vi "BNNN.vi"(11 "Variables and Memory in":T1 {"GFX" format="%02x"}) -> (3 "Variables and Memory out":T1 {"GFX" format="%02x"})   [LabVIEW 2021]
uses:
  Controls/ClusterF.ctl
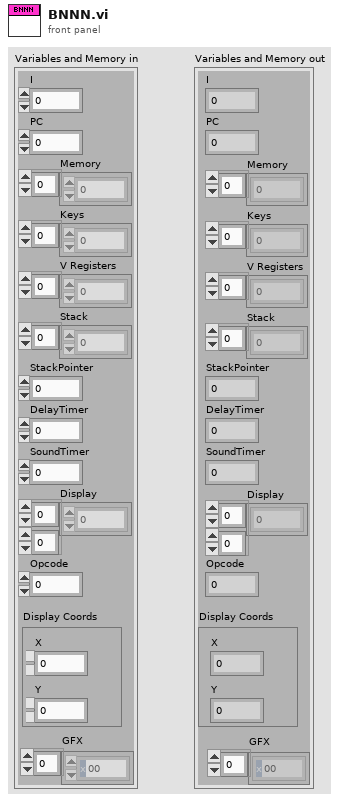
[diagram p1: front panel]
types:
  T1 = typedef "ClusterF.ctl" = cluster{"I":u16, "PC":u16, "Memory":u8[], "Keys":u8[], "V Registers":u8[], "Stack":u16[], "StackPointer":u16, "DelayTimer":u8, "SoundTimer":u8, "Display":u8[][], "Opcode":u16, "Display Coords":cluster{"X":u8, "Y":u8}, "GFX":u8[]}
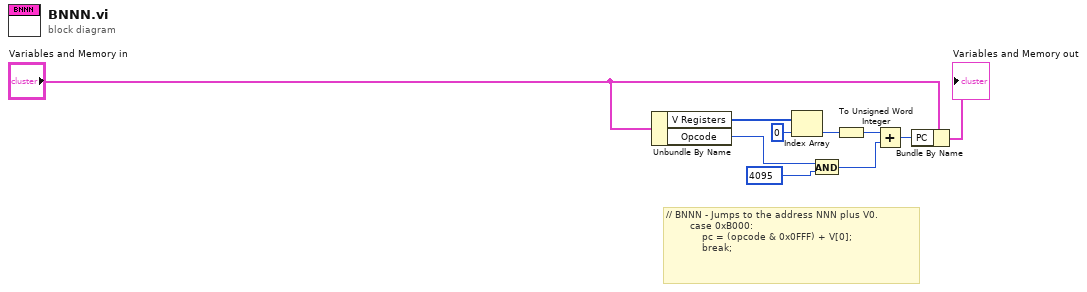
[diagram p0: block diagram]
diagram:
  # "// BNNN - Jumps to the address NNN plus V0.\n        case 0xB000:\n            pc = (opcode & 0x0FFF) + V[0];\n            break;"
  n1 = Unbundle By Name("Variables and Memory in") -> ("V Registers"=w3:u8[], "Opcode"=w1:u16)
  n2 = Index Array(array=w3, index=0) -> (element=w5:u8)
  n3 = And(x=w1, y=u16 4095) -> (x .and. y?=w6:u16)
  n4 = To Unsigned Word Integer(number=w5) -> (unsigned 16bit integer=w7:u16)
  n5 = Add(x=w7, y=w6) -> (x+y=w10:u16)
  n6 = Bundle By Name(cluster="Variables and Memory in", "PC"=w10) -> (→"Variables and Memory out":T1)
